vi "WPI_SolenoidGetBool.vi"(8 "error in (no error)":errorcluster, 11 "SolenoidDevRef":T1={"DevStatus"={"status"=FALSE, "code"=0, "source"=""}, "Pneumatics Control Module"=0, "Forward Solenoid Channel"=enum."Invalid", "Reverse Solenoid Channel"=enum."Invalid"}) -> (0 "error out":errorcluster, 2 "Value":bool, 3 "SolenoidDevRef":T1={"DevStatus"={"status"=FALSE, "code"=0, "source"=""}, "Pneumatics Control Module"=0, "Forward Solenoid Channel"=enum."Invalid", "Reverse Solenoid Channel"=enum."Invalid"})   [LabVIEW 2017]
doc: "Returns whether the solenoid you specify is On or Off.\n\nThis software is licensed. Open the labview\\readme\\WPI Robotics Library Open Source License.txt file for more information."
uses:
  <vilib>/Rock Robotics/WPI/Solenoid/WPI_SolenoidDevRef.ctl
  <vilib>/Rock Robotics/WPI/Solenoid/WPI_SolenoidChannel.ctl
  <vilib>/Rock Robotics/WPI/CAN/PCM/WPI_CAN_PCMGlobalOps.ctl
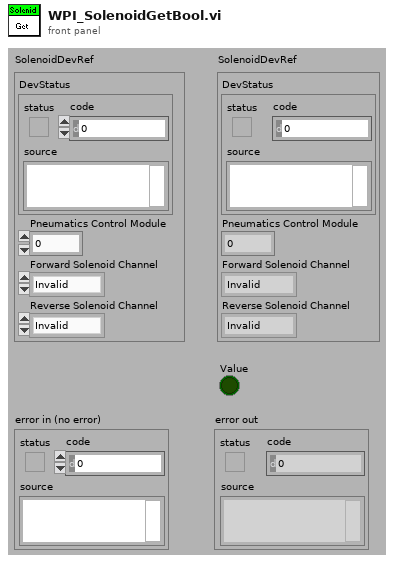
[diagram p1: front panel]
types:
  T1 = typedef "WPI_SolenoidDevRef.ctl" = cluster{"DevStatus":errorcluster, "Pneumatics Control Module":u8, "Forward Solenoid Channel":T2, "Reverse Solenoid Channel":T2}
  T2 = typedef "WPI_SolenoidChannel.ctl" = enum8{"Solenoid 0", "Solenoid 1", "Solenoid 2", "Solenoid 3", "Solenoid 4", "Solenoid 5", "Solenoid 6", "Solenoid 7", "Invalid"}
  T3 = typedef "WPI_CAN_PCMGlobalOps.ctl" = enum16{"Read For Send", "Write After Receive", "Set Solenoids", "Set Closed Loop", "Clear Sticky Faults", "Get All", "Write Error", "Write After Receive Blacklist", "Set Control Frame Rate"}
  T4 = cluster{"Solenoid Status":bool[], "Battery Voltage":dbl, "Solenoid Voltage":dbl, "Compressor Current":dbl, "CompressorEnabled":bool, "StickySolenoidFault":bool, "StickyCompressorFault":bool, "SolenoidFault":bool, "CompressorFault":bool, "HardwareFault":bool, "ClosedLoopStatus":bool, "PressureStatus":bool, "Module Enabled":bool, "ClosedLoopSuggestedOutput":bool, "CAN Error":errorcluster, "Sticky Solenoid Faults":bool[]}
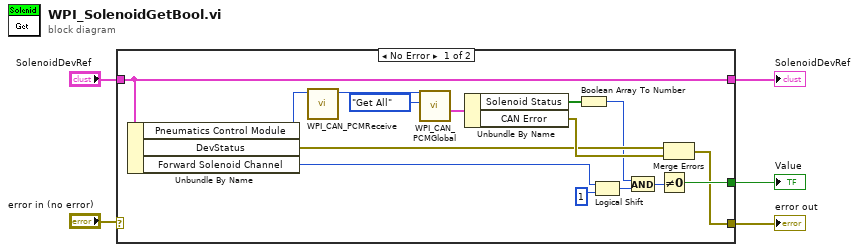
[diagram p0: block diagram]
diagram:
  n1 = case shown="No Error" "error in (no error)" {
    selector: "error in (no error)" -> [_ w22]
    tunnel: "SolenoidDevRef" -> [w6 w21]
    tunnel: [w12 w22] -> w3
    tunnel: [w6 w21] -> w2
    tunnel: [w16 _] -> w1
    frame No Error {
      n2 = Unbundle By Name(w6) -> ("Pneumatics Control Module"=w8:u8, "DevStatus"=w10:errorcluster, "Forward Solenoid Channel"=w19:T2)
      n3 = call <vilib>:"WPI_CAN_PCMReceive.vi"("Pneumatics Control Module (0)"=w8) -> ("Pneumatics Control Module Out"=w7:u8)  [unwired: 10 in]
      n4 = call <vilib>:"WPI_CAN_PCMGlobal.vi"("Operation"=WPI_CAN_PCMGlobalOps."Get All", "Pneumatics Control Module (0)"=w7) -> ("Get All"=w14:T4)  [unwired: 7 in, 2 out]
      n5 = Unbundle By Name(w14) -> ("Solenoid Status"=w13:bool[], "CAN Error"=w11:errorcluster)
      n6 = Boolean Array To Number(Boolean array=w13) -> (number=w9:u32)
      n7 = Logical Shift(y=w19, x=u8 1) -> (x << y=w18:u8)
      n8 = And(x=w9, y=w18) -> (x .and. y?=w17:u32)
      n9 = Not Equal To 0?(x=w17) -> (x != 0?=w16:bool)
      n10 = Merge Errors(w10, w11) -> (w12:errorcluster)
    }
    frame Error {
    }
  }
  "SolenoidDevRef" <- w2
  "error out" <- w3
  "Value" <- w1
